vi "Main Login.vi"() -> ()   [LabVIEW 2020]
uses:
  Support/Public/Polymorph/ini Ctrl_Str.vi
panel:
  out "Version":string
  in  "Password":string
  in  "User ID":string
  in  "확인":bool
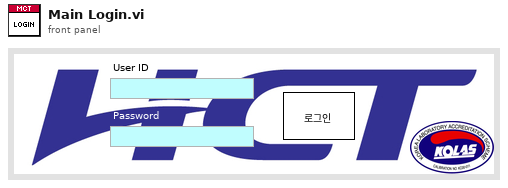
[diagram p1: front panel]
types:
  T1 = enum32{"Invalid", "Standard", "Closed", "Hidden", "Minimized", "Maximized"}
  T2 = enum32{"invalid app kind", "Development System", "Run Time System", "Student Edition", "Embedded LabVIEW", "Evaluation", "Custom"}
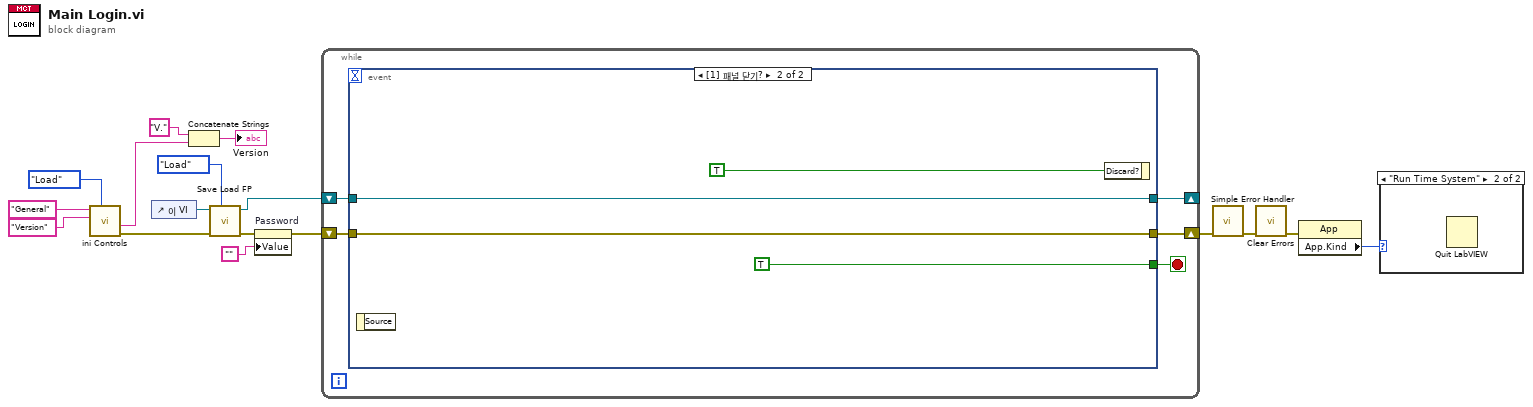
[diagram p0: block diagram]
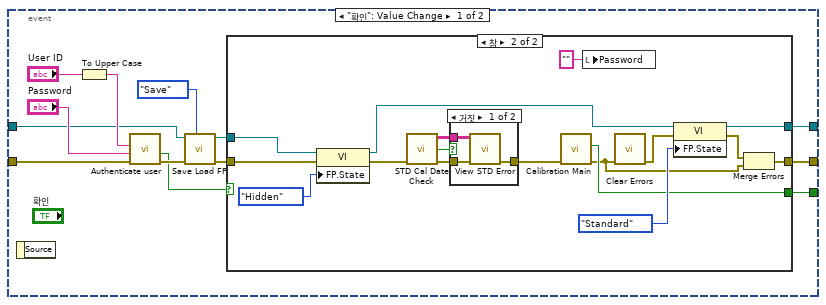
[diagram p3: hidden frame]
diagram:
  n1 = call-poly "ini Controls.vi"("Select"=enum16{"Save", "Load"}."Load", "키"="Version", "섹션"="General") -> ("에러 출력"=w7:errorcluster, "값"=w2:string)  [unwired: 6 in, 1 out]
  n2 = control-ref of="이 VI"() -> (w11:refnum<vi>)
  n3 = Concatenate Strings("V." ("문자열"), w2) -> (→"Version":string)
  n4 = call "Save Load FP.vi"("Menu"=enum16{"Save", "Load"}."Load", "error in"=w7, "VI 참조 번호"=w11) -> ("error out"=w17:errorcluster, "VI 참조 번호 out"=w10:refnum<vi>)  [unwired: 7 in]
  n5 = property on="Password" class="Str"(error in=w17, "Value"="" ("Password")) -> (error out=w15:errorcluster)  [unwired: 1 in, 1 out]
  n6 = while {
    shift-right: [w20] -> w12
    shift-left: w15 -> [w22]
    shift-right: [w18] -> _
    shift-left: w10 -> [w19]
    stop <- w21 stop-if-true
    n7 = event shown="[1] 패널 닫기?" {
      selector: _ -> [_ _]
      dyn-events: _ -> [_ _]
      timeout: _ -> [_ _]
      tunnel: w22 -> [w34 w61]
      tunnel: [w24 TRUE ("Verified?")] -> w21
      tunnel: [w28 w61] -> w20
      tunnel: w19 -> [w26 w59]
      tunnel: [w23 w59] -> w18
      event "확인": Value Change {
        n8 = event-data() -> ()  [unwired: 1 in, 1 out]
        n9 = To Upper Case(1:"User ID") -> (0:w31:string)
        n10 = call "Authenticate user.vi"("error in"=w34, "Password"="Password", "User ID"=w31) -> ("error out"=w33:errorcluster, "Verified?"=w27:bool)  [unwired: 7 in]
        n11 = call "Save Load FP.vi"("Menu"=enum16{"Save", "Load"}."Save", "error in"=w33, "VI 참조 번호"=w26) -> ("error out"=w29:errorcluster, "VI 참조 번호 out"=w25:refnum<vi>)  [unwired: 7 in]
        n12 = case shown="참" w27 {
          tunnel: w29 -> [w37 w42]
          tunnel: [w37 w40] -> w28
          tunnel: w25 -> [w36 w49]
          tunnel: [_ w48] -> w24
          tunnel: [w36 w47] -> w23
          frame False {
          }
          frame True {
            n13 = property class="VI"(reference=w49, error in=w42, "FP.State"=T1."Hidden" ("프런트패널 윈도우:상태")) -> (reference out=w50:refnum<vi>, error out=w41:errorcluster)
            n14 = call "STD Cal Date Check.vi"("에러 입력"=w41) -> ("error out"=w45:errorcluster, "비어있음?"=w46:bool, "Data"=w44:string[][])  [unwired: 8 in]
            n15 = case shown="거짓" w46 {
              tunnel: w45 -> [w57 w58]
              tunnel: [w56 w58] -> w43
              tunnel: w44 -> [w55 _]
              frame False {
                n16 = call "View STD Error.vi"("error in"=w57, "Data"=w55) -> ("error out"=w56:errorcluster)  [unwired: 9 in]
              }
              frame True {
              }
            }
            n17 = call "Calibration Main.vi"("error in"=w43) -> ("error out"=w38:errorcluster, "종료?"=w48:bool)  [unwired: 9 in]
            n18 = local write "Password"("" ("Password")) -> ()
            n19 = call <vilib>:"Clear Errors.vi"("error in (no error)"=w38) -> ("error out"=w53:errorcluster)  [unwired: 5 in, 1 out]
            n20 = property class="VI"(reference=w50, error in=w53, "FP.State"=T1."Standard" ("프런트패널 윈도우:상태")) -> (reference out=w47:refnum<vi>, error out=w39:errorcluster)
            n21 = Merge Errors(w39, w38) -> (w40:errorcluster)
          }
        }
      }
      event Panel Close? {
        n22 = event-data() -> ()  [unwired: 1 in, 1 out]
        n23 = event-data("Discard?"=TRUE ("버림?")) -> ()  [unwired: 1 in, 1 out]
      }
    }
  }
  n24 = call <vilib>:"Simple Error Handler.vi"("error in (no error)"=w12) -> ("error out"=w8:errorcluster)  [unwired: 4 in, 4 out]
  n25 = call <vilib>:"Clear Errors.vi"("error in (no error)"=w8) -> ("error out"=w9:errorcluster)  [unwired: 5 in, 1 out]
  n26 = property class="App"(error in=w9) -> ("App.Kind"=w13:T2)  [unwired: 1 in, 2 out]
  n27 = case shown="\"Run Time System\"" w13 {
    frame Default {
    }
    frame "Run Time System" {
      n28 = Quit LabVIEW() -> ()  [unwired: 1 in]
    }
  }
